vi "response.To JSON String.vi"(8 "error in (no error)":errorcluster, 11 "Response in":refnum<class "Response.lvclass">) -> (0 "error out":errorcluster, 2 "JSON String":string, 3 "Response out":refnum<class "Response.lvclass">)   [LabVIEW 2016, in "Response.lvclass"]
uses:
  Response.lvclass
  <vilib>/NI/JSON Support for LabVIEW/JSON Value/JSON Value.lvclass
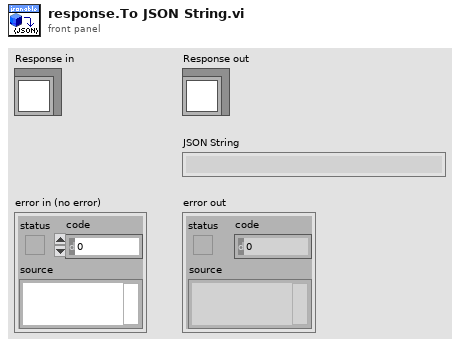
[diagram p1: front panel]
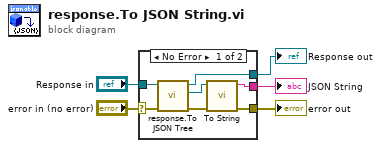
[diagram p0: block diagram]
diagram:
  n1 = case shown="No Error" "error in (no error)" {
    selector: "error in (no error)" -> [w11 w14]
    tunnel: [w7 w14] -> w4
    tunnel: [w10 w13] -> w2
    tunnel: "Response in" -> [w12 w13]
    tunnel: [w8 _] -> w1
    frame No Error {
      n2 = call "response.To JSON Tree.vi"("error in (no error)"=w11, "Response in"=w12) -> ("error out"=w6:errorcluster, "JSON Value out"=w9:refnum<class "JSON Value.lvclass">, "Response out"=w10:refnum<class "Response.lvclass">)  [unwired: 7 in]
      n3 = call <vilib>:"To String.vi"("error in (no error)"=w6, "JSON Value in"=w9) -> ("error out"=w7:errorcluster, "String"=w8:string)  [unwired: 8 in]
    }
    frame Error {
    }
  }
  "error out" <- w4
  "Response out" <- w2
  "JSON String" <- w1
